vi "DAQSettingsDialog.vi"(8 "error in (no error)":errorcluster, 11 "Acquisition Settings In":T1) -> (0 "error out":errorcluster, 2 "UI Refresh Needed?":bool, 3 "Acquisition Settings Out":T1)   [LabVIEW 2014]
uses:
  controls/TriggerMode.ctl
  controls/DAQSettings.ctl
panel:
  in  "Cancel Button":bool
  in  "OK Button":bool
  in  "Trigger":T2
  in  "Repetition":dbl
  in  "Pixel Number":dbl
  # "DAQ settings"
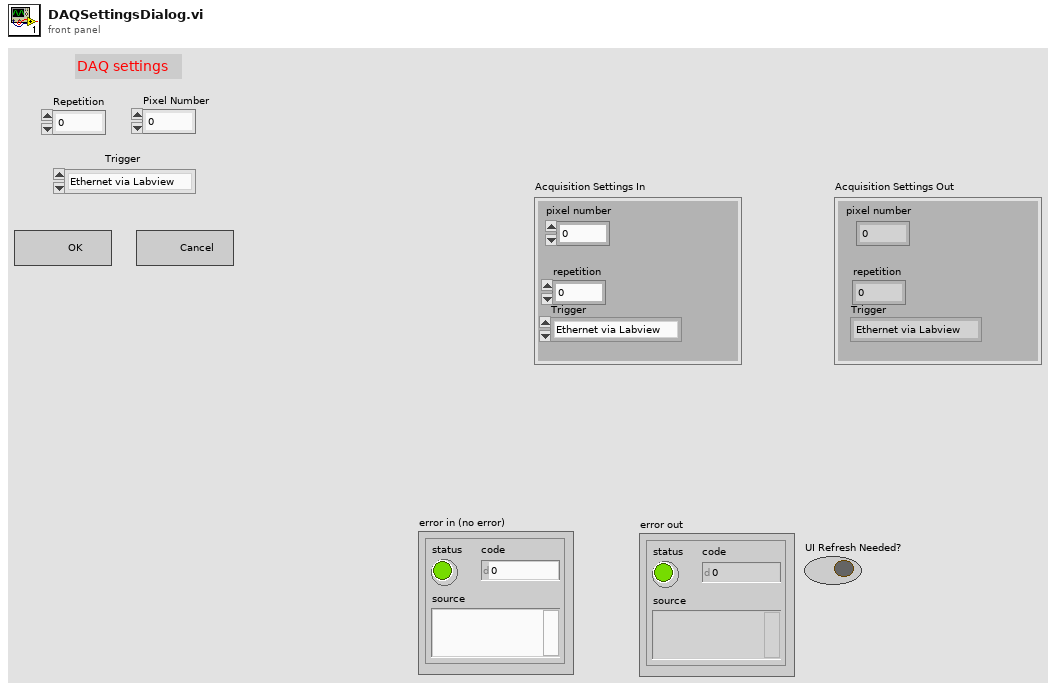
[diagram p1: front panel]
types:
  T1 = typedef "DAQSettings.ctl" = cluster{"pixel number":u32, "repetition":u32, "Trigger":T2}
  T2 = typedef "TriggerMode.ctl" = enum16{"Ethernet via Labview", "SMA (1.8V)"}
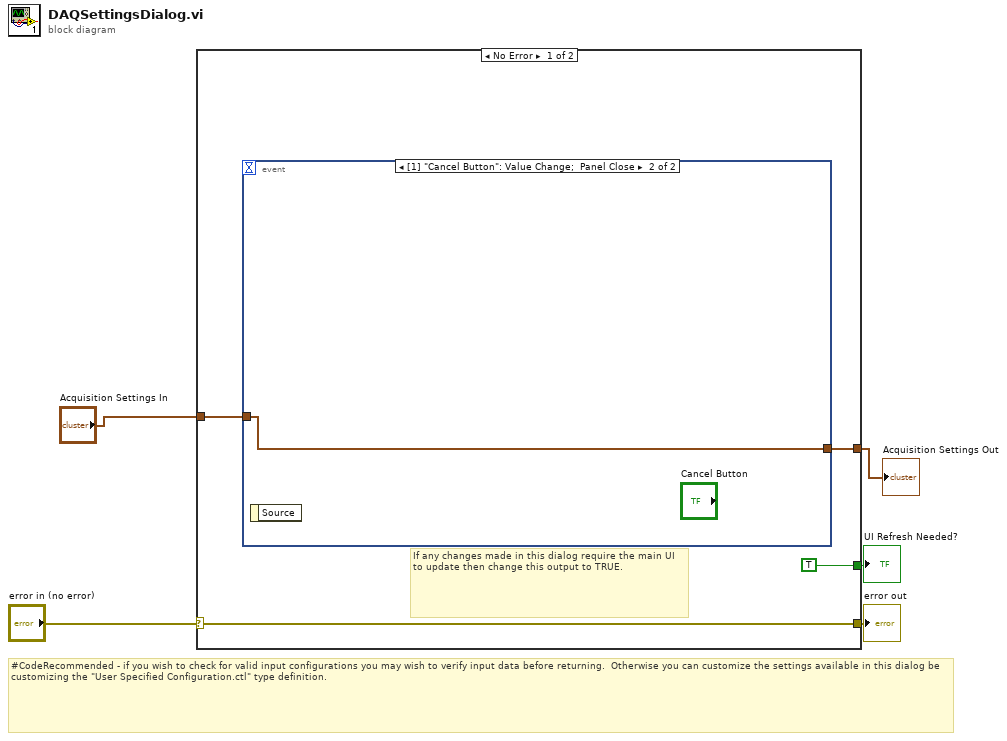
[diagram p0: block diagram]
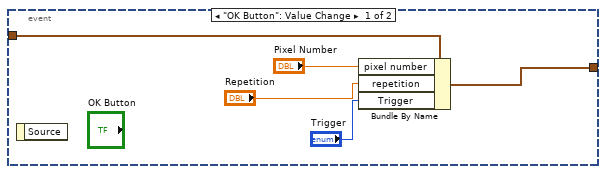
[diagram p2: hidden frame]
diagram:
  # "#CodeRecommended - if you wish to check for valid input configurations you may wish to verify input data before returning.  Otherwise you can customize the settings available in this dialog be customizing the \"User Specified Configuration.ctl\" type definition."
  n1 = case shown="No Error" "error in (no error)" {
    selector: "error in (no error)" -> [w9 w17]
    tunnel: [w9 w17] -> w4
    tunnel: [TRUE ("UI Refresh Needed?") _] -> w3
    tunnel: "Acquisition Settings In" -> [w7 w16]
    tunnel: [w6 w16] -> w1
    frame No Error {
      # "If any changes made in this dialog require the main UI to update then change this output to TRUE."
      n2 = event shown="[1] \"Cancel Button\": Value Change;  Panel Close" {
        selector: _ -> [_ _]
        dyn-events: _ -> [_ _]
        timeout: _ -> [_ _]
        tunnel: w7 -> [w14 w15]
        tunnel: [w13 w15] -> w6
        event "OK Button": Value Change {
          n3 = event-data() -> ()  [unwired: 1 in, 1 out]
          n4 = Bundle By Name(cluster=w14, "pixel number"="Pixel Number", "repetition"="Repetition", "Trigger"="Trigger") -> (w13:T1)
        }
        event "Cancel Button": Value Change; Panel Close {
          n5 = event-data() -> ()  [unwired: 1 in, 1 out]
        }
      }
    }
    frame Error {
    }
  }
  "UI Refresh Needed?" <- w3
  "error out" <- w4
  "Acquisition Settings Out" <- w1
